vi "Replace Compiled Settings Cluster Control.vi"(6 "Position:Top":i32=248, 8 "error in":errorcluster, 10 "ctl path":path, 11 "VI in":refnum<vi>) -> (0 "error out":errorcluster)   [LabVIEW 2026, in "NIVS_CDEW_MetaDataObj.lvclass"]
uses:
  NIVS_CDEW_MetaDataObj.lvclass
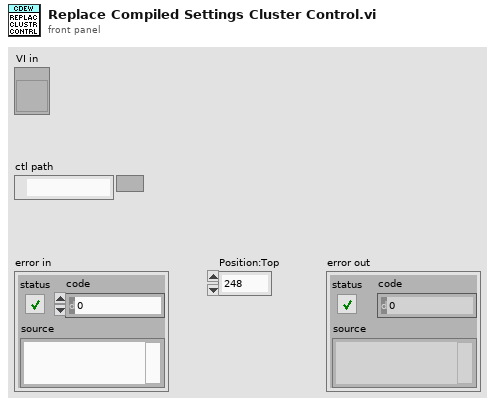
[diagram p1: front panel]
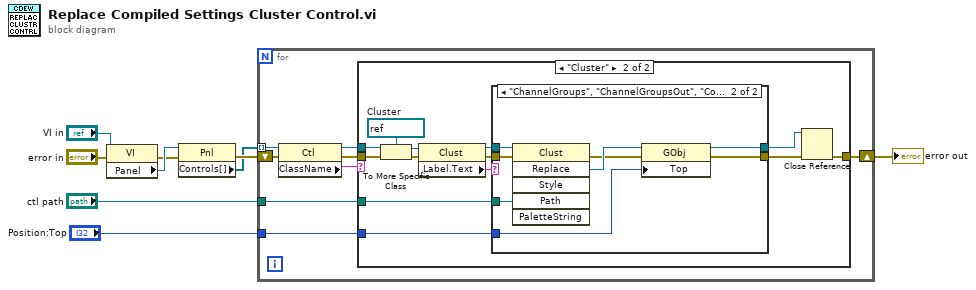
[diagram p0: block diagram]
diagram:
  n1 = property class="VI"(reference="VI in", error in="error in") -> (error out=w3:errorcluster, "Panel"=w4:refnum<vi>)  [unwired: 1 out]
  n2 = property class="Pnl"(reference=w4, error in=w3) -> (error out=w7:errorcluster, "Controls[]"=w5:refnum<vi>[])  [unwired: 1 out]
  n3 = for {
    tunnel: w5 -> [w17] mode=indexing
    tunnel: "ctl path" -> [w13]
    shift-right: [w12] -> w8
    shift-left: w7 -> [w11]
    tunnel: "Position:Top" -> [w10]
    n4 = property class="Ctl"(reference=w17, error in=w11) -> (reference out=w14:refnum<vi>, error out=w15:errorcluster, "ClassName"=w16:string)
    n5 = case shown="\"Cluster\"" w16 {
      tunnel: w15 -> [w18 w31]
      tunnel: w14 -> [_ w30]
      tunnel: w13 -> [_ w23]
      tunnel: [w18 w20] -> w12
      tunnel: w10 -> [_ w19]
      frame Default {
      }
      frame "Cluster" {
        w29 = refnum<vi> refnum  # Cluster
        n6 = To More Specific Class(target class=w29, reference=w30, error in=w31) -> (specific class reference=w27:refnum<vi>, error out=w28:errorcluster)
        n7 = property class="Clust"(reference=w27, error in=w28) -> (reference out=w24:refnum<vi>, error out=w25:errorcluster, "Label.Text"=w26:string)
        n8 = case shown="\"ChannelGroups\", \"ChannelGroupsOut\", \"CompiledSettings\", \"CompiledSettingsOut\"" w26 {
          tunnel: w25 -> [w32 w40]
          tunnel: w24 -> [w33 w39]
          tunnel: w23 -> [_ w38]
          tunnel: [w33 w37] -> w21
          tunnel: [w32 w35] -> w22
          tunnel: w19 -> [_ w34]
          frame "not a typedef", Default {
          }
          frame "ChannelGroups", "ChannelGroupsOut", "CompiledSettings", "CompiledSettingsOut" {
            n9 = invoke class="Clust" method="Replace"(reference=w39, error in=w40, "Path"=w38) -> (error out=w36:errorcluster, "Replace"=w37:refnum<vi>)  [unwired: 3 in, 4 out]
            n10 = property class="GObj"(reference=w37, error in=w36, "Top"=w34) -> (error out=w35:errorcluster)  [unwired: 1 out]
          }
        }
        n11 = Close Reference(reference=w21, error in (no error)=w22) -> (error out=w20:errorcluster)
      }
    }
  }
  "error out" <- w8
